vi "BatchProcessWindow_lvcicd.vi"(6 "FP(T)":bool=TRUE, 7 "VI Refnum":refnum<vi>, 8 "error in (no error)":errorcluster, 9 "silence mode(F)":bool, 11 "paths":path[](array[path])) -> (0 "error out":errorcluster, 3 "Array":string[][](array[string]))   [LabVIEW 2014, in "_lvcicd_support.lvlib"]
uses:
  _lvcicd_support.lvlib
panel:
  out "VIREF":refnum<vi>
  out "Information":i32(listbox)
  in  "Terminal?":bool
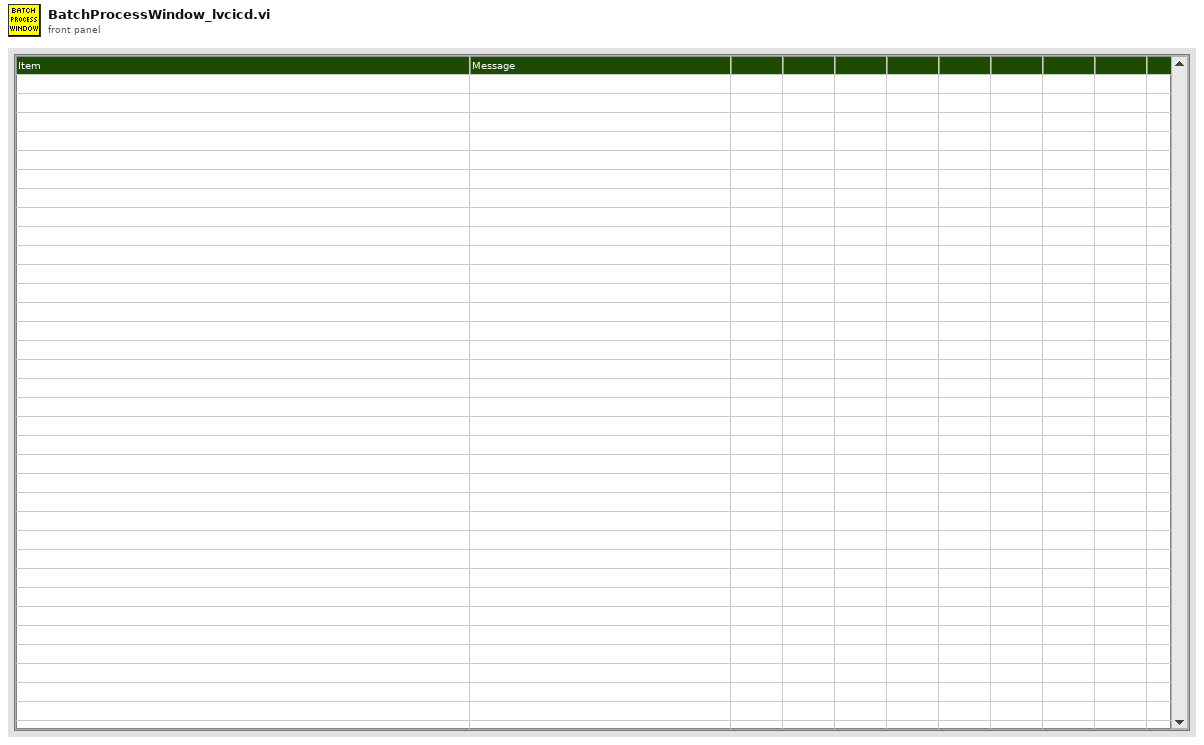
[diagram p1: front panel]
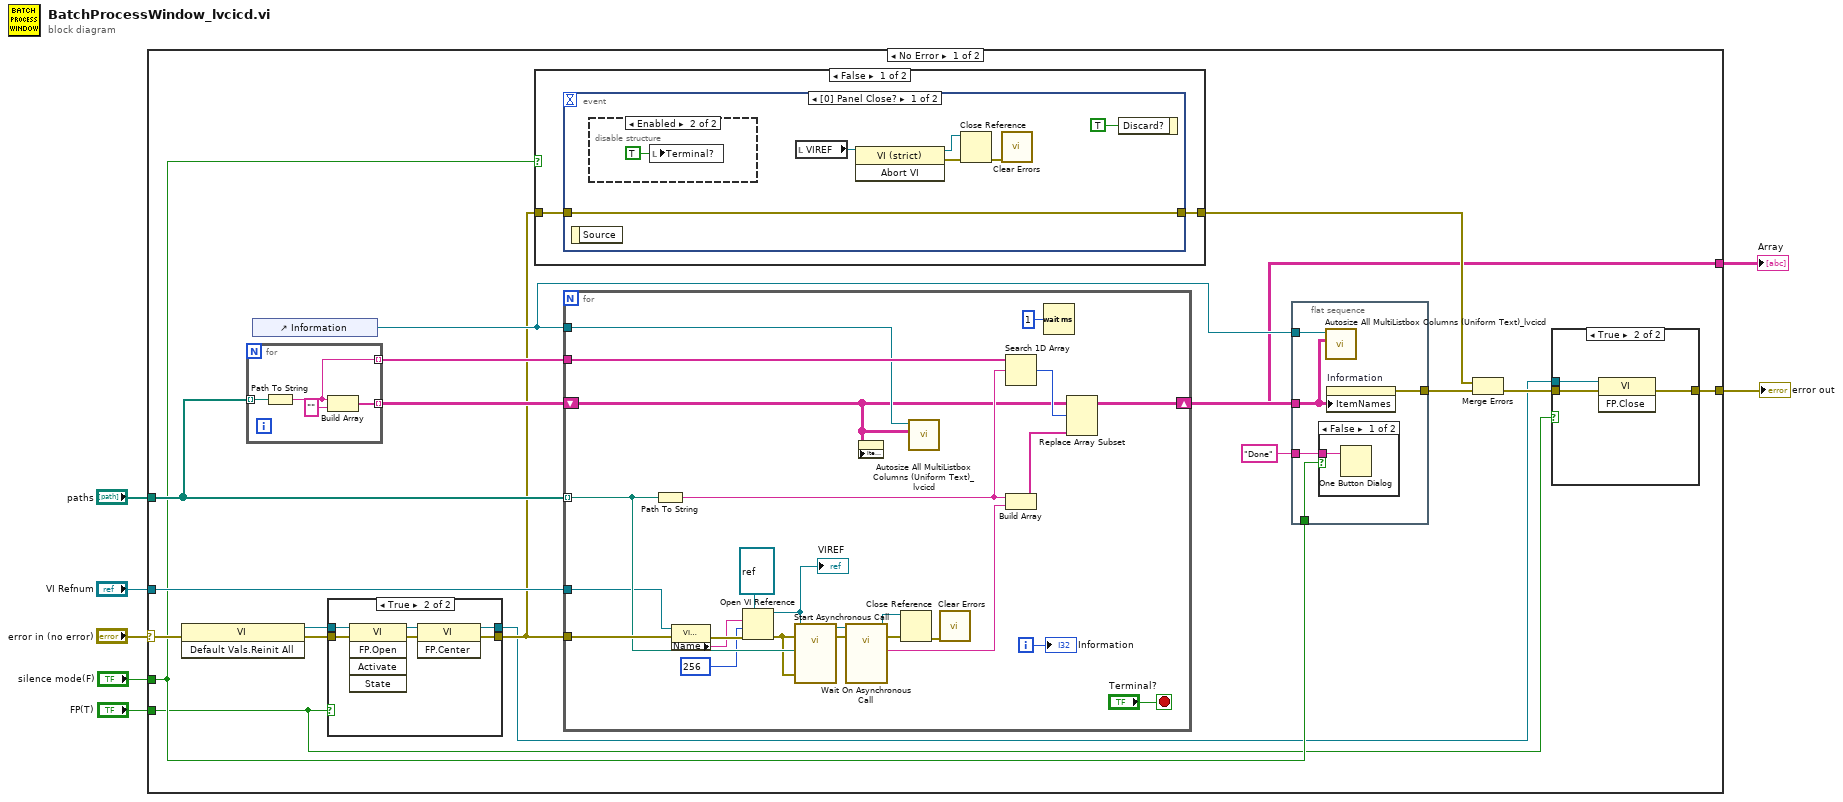
[diagram p0: block diagram]
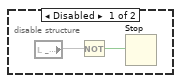
[diagram p3: hidden frame]
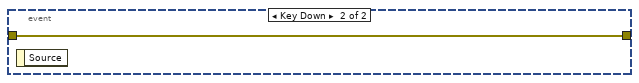
[diagram p4: hidden frame]
diagram:
  n1 = case shown="No Error" "error in (no error)" {
    selector: "error in (no error)" -> [w21 w87]
    tunnel: [w10 w87] -> w5
    tunnel: "paths" -> [w22 _]
    tunnel: "VI Refnum" -> [w20 _]
    tunnel: "silence mode(F)" -> [w13 _]
    tunnel: "FP(T)" -> [w8 _]
    tunnel: [w12 _] -> w1
    frame No Error {
      n2 = invoke class="VI" method="Default Vals.Reinit All"(error in=w21) -> (reference out=w15:refnum<vi>, error out=w19:errorcluster)  [unwired: 2 in, 1 out]
      n3 = for {
        tunnel: w22 -> [w59] mode=indexing
        tunnel: [w61] -> w26 mode=indexing
        tunnel: [w58] -> w25 mode=indexing
        n4 = Path To String(path=w59) -> (string=w58:string)
        n5 = Build Array(w58, "" ("element")) -> (w61:string[])
      }
      n6 = control-ref of="Information"() -> (w18:refnum<vi>)
      n7 = case shown="True" w8 {
        tunnel: w19 -> [w45 w51]
        tunnel: [w45 w48] -> w16
        tunnel: w15 -> [w44 w49]
        tunnel: [w44 w46] -> w9
        frame False {
        }
        frame True {
          n8 = invoke class="VI" method="FP.Open"(reference=w49, error in=w51) -> (reference out=w47:refnum<vi>, error out=w50:errorcluster)  [unwired: 3 in, 3 out]
          n9 = invoke class="VI" method="FP.Center"(reference=w47, error in=w50) -> (reference out=w46:refnum<vi>, error out=w48:errorcluster)  [unwired: 1 in, 1 out]
        }
      }
      n10 = case shown="False" w13 {
        tunnel: [w32 w43] -> w17
        tunnel: w16 -> [w31 w43]
        frame False {
          n11 = event shown="[0] Panel Close?" {
            selector: _ -> [_ _]
            dyn-events: _ -> [_ _]
            timeout: _ -> [_ _]
            tunnel: w31 -> [w37 w42]
            tunnel: [w37 w42] -> w32
            event Panel Close? {
              n12 = event-data() -> ()  [unwired: 1 in, 1 out]
              n13 = disable-structure shown="Enabled" {
                frame Disabled {
                  n14 = local read item#-1() -> (w40)
                  n15 = Not(x=w40) -> (.not. x?=w39:bool)
                  n16 = Stop(stop? (T)=w39) -> ()
                }
                frame Enabled {
                  n17 = local write "Terminal?"(TRUE ("Terminal?")) -> ()
                }
              }
              n18 = local read "VIREF"() -> (w34:refnum<vi>)
              n19 = invoke class="VI (strict)" method="Abort VI"(reference=w34) -> (reference out=w36:refnum<vi>, error out=w35:errorcluster)  [unwired: 2 in, 1 out]
              n20 = Close Reference(reference=w36, error in (no error)=w35) -> (error out=w33:errorcluster)
              n21 = call <vilib>:"Clear Errors.vi"("error in (no error)"=w33) -> ()  [unwired: 5 in, 2 out]
              n22 = event-data("Discard?"=TRUE) -> ()  [unwired: 1 in, 1 out]
            }
            event Key Down {
              n23 = event-data() -> ()  [unwired: 1 in, 1 out]
            }
          }
        }
        frame True {
        }
      }
      n24 = for {
        tunnel: w22 -> [w79] mode=indexing
        tunnel: w16 -> [w85]
        shift-right: [w83] -> w24
        shift-left: w26 -> [w62]
        tunnel: w25 -> [w84]
        tunnel: w20 -> [w77]
        tunnel: w18 -> [w63]
        i -> [w80]
        stop <- "Terminal?" stop-if-true
        n25 = Path To String(path=w79) -> (string=w78:string)
        n26 = property class="VI (strict)"(reference=w77, error in=w85) -> (error out=w73:errorcluster, "Name"=w72:string)  [unwired: 1 out]
        n27 = Open VI Reference(type specifier VI Refnum (for type only)=refnum<vi> refnum, vi path=w72, options=256, error in (no error)=w73) -> (vi reference=w70:refnum<vi>, error out=w74:errorcluster)  [unwired: 2 in]
        "VIREF" <- w70
        n28 = call-by-ref "Start Asynchronous Call"(reference=w70, error in=w74, 8:"error in (no error)"=w74, "Path"=w79) -> (reference out=w68:refnum<vi>, error out=w67:errorcluster)  [unwired: 9 in, 1 out]
        n29 = call-by-ref "Wait On Asynchronous Call"(reference=w68, error in=w67) -> (reference out=w65:refnum<vi>, error out=w66:errorcluster, "f"=w86:string)  [unwired: 11 in]
        n30 = property on="Information" class="MCListbox (strict)"("ItemNames"=w62) -> ()  [unwired: 2 in, 2 out]
        n31 = Close Reference(reference=w65, error in (no error)=w66) -> (error out=w64:errorcluster)
        n32 = call "Autosize All MultiListbox Columns (Uniform Text)_lvcicd.vi"("Array"=w62, "Control in"=w63) -> ()  [unwired: 8 in, 2 out]
        n33 = call <vilib>:"Clear Errors.vi"("error in (no error)"=w64) -> ()  [unwired: 5 in, 2 out]
        n34 = Search 1D Array(1D array=w84, element=w78) -> (index of element=w82:i32)  [unwired: 1 in]
        n35 = Build Array(w78, w86) -> (w81:string[])
        n36 = Wait (ms)(milliseconds to wait=u32 1) -> ()  [unwired: 1 out]
        n37 = Replace Array Subset(array=w62, new element=w81, index (row)=w82) -> (w83:string[][])  [unwired: 1 in]
        "Information" <- w80
      }
      n38 = flat-sequence {
        tunnel: w24 -> [w52]
        tunnel: [w56] -> w23
        tunnel: w18 -> [w55]
        tunnel: "Done" ("message") -> [w54]
        tunnel: w13 -> [w53]
        tunnel: [w52] -> w12
        frame #0 {
          n39 = case shown="False" w53 {
            tunnel: w54 -> [w57 _]
            frame False {
              n40 = One Button Dialog(message=w57) -> ()  [unwired: 1 in, 1 out]
            }
            frame True {
            }
          }
          n41 = call "Autosize All MultiListbox Columns (Uniform Text)_lvcicd.vi"("Array"=w52, "Control in"=w55) -> ()  [unwired: 8 in, 2 out]
          n42 = property on="Information" class="MCListbox (strict)"("ItemNames"=w52) -> (error out=w56:errorcluster)  [unwired: 2 in, 1 out]
        }
      }
      n43 = Merge Errors(w17, w23) -> (w11:errorcluster)
      n44 = case shown="True" w8 {
        tunnel: w11 -> [w27 w30]
        tunnel: [w27 w29] -> w10
        tunnel: w9 -> [_ w28]
        frame False {
        }
        frame True {
          n45 = invoke class="VI" method="FP.Close"(reference=w28, error in=w30) -> (error out=w29:errorcluster)  [unwired: 1 in, 2 out]
        }
      }
    }
    frame Error {
    }
  }
  "error out" <- w5
  "Array" <- w1
